vi "dfd_Left Multiply Diagonal Matrix.vi"   [LabVIEW 2017, in "NI_DigFilter_Design.lvlib"]
uses:
  <vilib>/addons/Digital Filter Design/NI_DigFilter_Design.lvlib
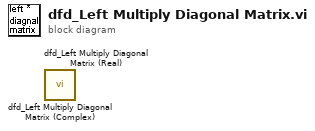
[diagram p0: block diagram]
diagram:
  n1 = call <vilib>:"dfd_Left Multiply Diagonal Matrix (Complex).vi"() -> ()  [unwired: 10 in, 2 out]
  n2 = call <vilib>:"dfd_Left Multiply Diagonal Matrix (Real).vi"() -> ()  [unwired: 10 in, 2 out]
